vi "Stop.vi"(8 "error in (no error)":errorcluster, 11 "FitterBase in":refnum<class "FitterBase.lvclass">) -> (0 "error out":errorcluster, 3 "FitterBase out":refnum<class "FitterBase.lvclass">)   [LabVIEW 2018, in "AnalysisPlugins.lvlib" / "FitterBase.lvclass"]
uses:
  FitterBase.lvclass
  C:/projects/ICDAS/NistPluggableModules/Analysis/AnalysisPlugins/AnalysisPluginBaseClass/AnalysisPluginsBase.lvclass
  AnalysisPluginBaseClass/Typedefs/clSensorData.ctl
  AnalysisPluginBaseClass/AnalysisPluginsBase.lvclass/AnalysisPluginsBase.ctl
  AnalysisPluginBaseClass/Accessors/Read SensorQue.vi
  AnalysisPluginBaseClass/Accessors/Write SensorQue.vi
  AnalysisPluginBaseClass/AnalysisPluginsBase.lvclass
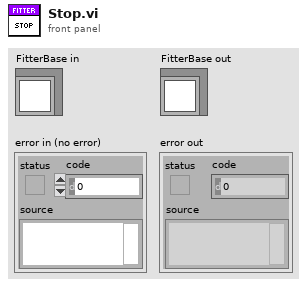
[diagram p1: front panel]
types:
  T1 = typedef "SensorQueue.ctl" = refnum<queue>
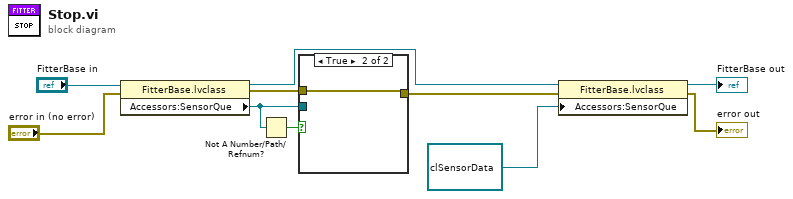
[diagram p0: block diagram]
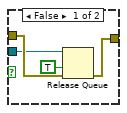
[diagram p2: hidden frame]
diagram:
  n1 = property class="FitterBase.lvclass"(reference="FitterBase in", error in="error in (no error)") -> (reference out=w7:refnum<class "FitterBase.lvclass">, error out=w8:errorcluster, "Accessors:SensorQue"=w2:T1)
  n2 = Not A Number/Path/Refnum?(number/path/refnum=w2) -> (NaN/Path/Refnum?=w1:bool)
  n3 = case shown="True" w1 {
    tunnel: w8 -> [w13 w15]
    tunnel: [w12 w15] -> w5
    tunnel: w2 -> [w11 _]
    frame False {
      n4 = Release Queue(queue=w11, force destroy? (F)=TRUE, error in (no error)=w13) -> (error out=w12:errorcluster)  [unwired: 2 out]
    }
    frame True {
    }
  }
  n5 = property class="FitterBase.lvclass"(reference=w7, error in=w5, "Accessors:SensorQue"=refnum<queue> refnum ("SensorQue")) -> (reference out=→"FitterBase out":refnum<class "FitterBase.lvclass">, error out=→"error out":errorcluster)
